vi "WPI_ADI_IMU_IMUAccumulation.vi"(1 "Input Data":T1) -> (0 "Output Data":T1)   [LabVIEW 2015, in "FRC ADI MXP IMU.lvlib"]
uses:
  FRC ADI MXP IMU.lvlib
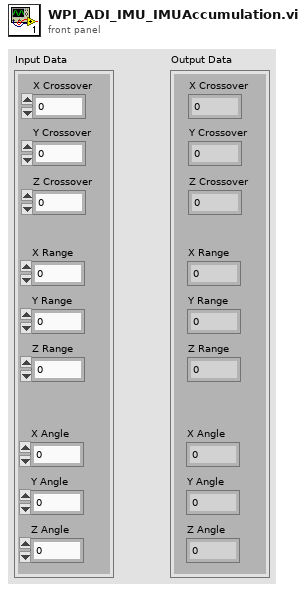
[diagram p1: front panel]
types:
  T1 = cluster{"X Crossover":dbl, "Y Crossover":dbl, "Z Crossover":dbl, "X Range":dbl, "Y Range":dbl, "Z Range":dbl, "X Angle":dbl, "Y Angle":dbl, "Z Angle":dbl}
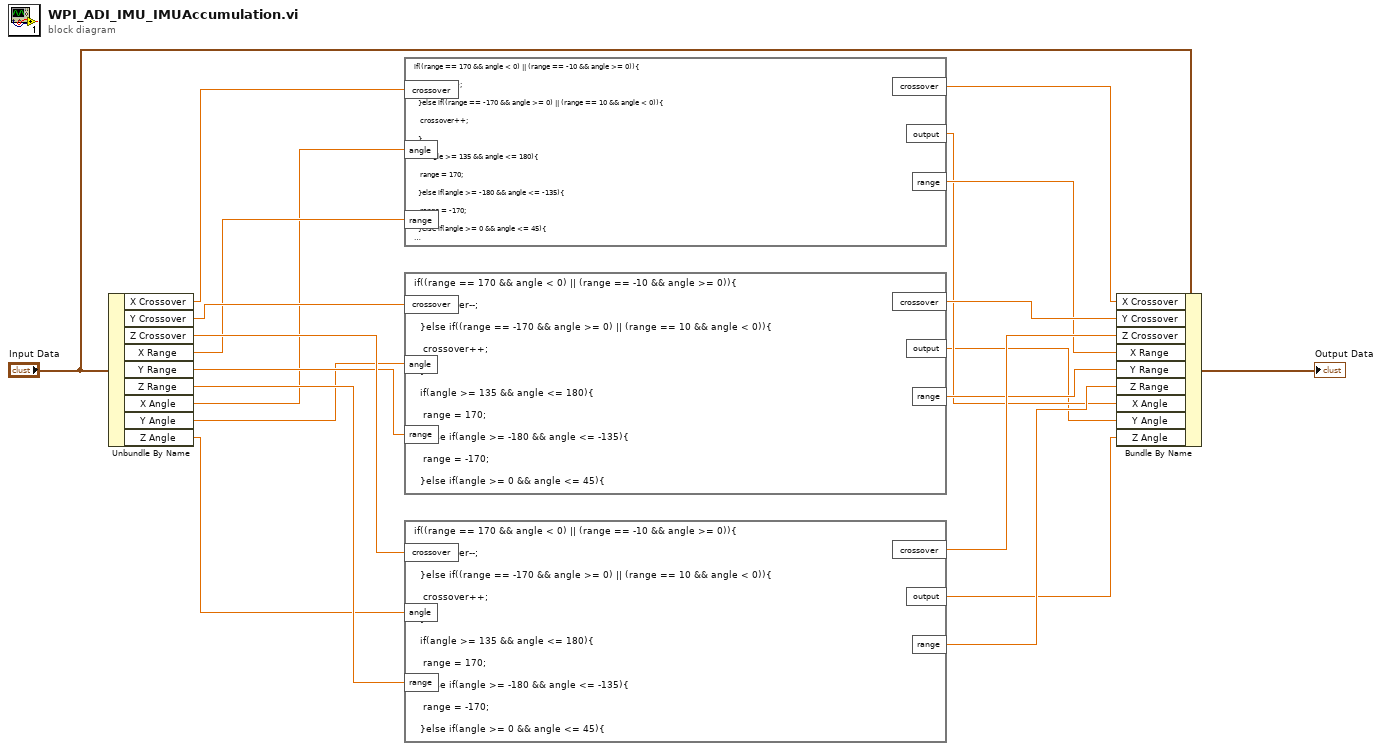
[diagram p0: block diagram]
diagram:
  n1 = Unbundle By Name("Input Data") -> ("X Crossover"=w20:dbl, "Y Crossover"=w19:dbl, "Z Crossover"=w18:dbl, "X Range"=w17:dbl, "Y Range"=w16:dbl, "Z Range"=w15:dbl, "X Angle"=w14:dbl, "Y Angle"=w13:dbl, "Z Angle"=w12:dbl)
  n2 = formula code="if((range == 170 && angle < 0) || (range == -10 && angle >= 0)){\n\t\t\n\t\t\tcrossover--;\n\t\t\t\n\t\t}else if((range == -170 && angle >= 0) || (range == 10 && angle < 0)){\n\t\t\n\t\t\tcrossover++;\n\t\t\t\n\t\t}\n\t\t\t\n\t\tif(angle >= 135 && angle <= 180){\n\t\t\n\t\t\trange = 170;\n\t\t\t\n\t\t}else if(angle >= -180 && angle <= -135){\n\t\t\n\t\t\trange = -170;\n\t\t\t\n\t\t}else if(angle >= 0 && angle <= 45){\n\t\t\n\t\t\trange = 10;\n\t\t\t\n\t\t}else if(angle >= -45 && angle <= 0){\n\t\t\n\t\t\trange = -10;\n\t\t\t\n\t\t}else{\n\t\t\n\t\t\trange = 0;\n\t\t\t\n\t\t}\n\t\t\n\t\tif(crossover != 0){\n\t\t\n\t\t\tif(angle < 0){\n\t\t\t\n\t\t\t\toutput = abs(180 + angle) + (-180 * crossover);\n\t\t\t\n\t\t\t}else{\n\t\t\n\t\t\t\toutput = abs(0 - angle) + (-180 * crossover);\n\t\t\n\t\t\t}\n\t\t\n\t\t}else{\n\t\t\n\t\t\toutput = angle;\n\t\t\n\t\t}"("crossover"=w20, "angle"=w14, "range"=w17) -> ("crossover"=w10:dbl, "output"=w4:dbl, "range"=w7:dbl)
  n3 = formula code="if((range == 170 && angle < 0) || (range == -10 && angle >= 0)){\n\t\t\n\t\t\tcrossover--;\n\t\t\t\n\t\t}else if((range == -170 && angle >= 0) || (range == 10 && angle < 0)){\n\t\t\n\t\t\tcrossover++;\n\t\t\t\n\t\t}\n\t\t\t\n\t\tif(angle >= 135 && angle <= 180){\n\t\t\n\t\t\trange = 170;\n\t\t\t\n\t\t}else if(angle >= -180 && angle <= -135){\n\t\t\n\t\t\trange = -170;\n\t\t\t\n\t\t}else if(angle >= 0 && angle <= 45){\n\t\t\n\t\t\trange = 10;\n\t\t\t\n\t\t}else if(angle >= -45 && angle <= 0){\n\t\t\n\t\t\trange = -10;\n\t\t\t\n\t\t}else{\n\t\t\n\t\t\trange = 0;\n\t\t\t\n\t\t}\n\t\t\n\t\tif(crossover != 0){\n\t\t\n\t\t\tif(angle < 0){\n\t\t\t\n\t\t\t\toutput = abs(180 + angle) + (-180 * crossover);\n\t\t\t\n\t\t\t}else{\n\t\t\n\t\t\t\toutput = abs(0 - angle) + (-180 * crossover);\n\t\t\n\t\t\t}\n\t\t\n\t\t}else{\n\t\t\n\t\t\toutput = angle;\n\t\t\n\t\t}"("crossover"=w19, "angle"=w13, "range"=w16) -> ("crossover"=w9:dbl, "output"=w2:dbl, "range"=w6:dbl)
  n4 = formula code="if((range == 170 && angle < 0) || (range == -10 && angle >= 0)){\n\t\t\n\t\t\tcrossover--;\n\t\t\t\n\t\t}else if((range == -170 && angle >= 0) || (range == 10 && angle < 0)){\n\t\t\n\t\t\tcrossover++;\n\t\t\t\n\t\t}\n\t\t\t\n\t\tif(angle >= 135 && angle <= 180){\n\t\t\n\t\t\trange = 170;\n\t\t\t\n\t\t}else if(angle >= -180 && angle <= -135){\n\t\t\n\t\t\trange = -170;\n\t\t\t\n\t\t}else if(angle >= 0 && angle <= 45){\n\t\t\n\t\t\trange = 10;\n\t\t\t\n\t\t}else if(angle >= -45 && angle <= 0){\n\t\t\n\t\t\trange = -10;\n\t\t\t\n\t\t}else{\n\t\t\n\t\t\trange = 0;\n\t\t\t\n\t\t}\n\t\t\n\t\tif(crossover != 0){\n\t\t\n\t\t\tif(angle < 0){\n\t\t\t\n\t\t\t\toutput = abs(180 + angle) + (-180 * crossover);\n\t\t\t\n\t\t\t}else{\n\t\t\n\t\t\t\toutput = abs(0 - angle) + (-180 * crossover);\n\t\t\n\t\t\t}\n\t\t\n\t\t}else{\n\t\t\n\t\t\toutput = angle;\n\t\t\n\t\t}"("crossover"=w18, "angle"=w12, "range"=w15) -> ("crossover"=w8:dbl, "output"=w3:dbl, "range"=w5:dbl)
  n5 = Bundle By Name(cluster="Input Data", "X Crossover"=w10, "Y Crossover"=w9, "Z Crossover"=w8, "X Range"=w7, "Y Range"=w6, "Z Range"=w5, "X Angle"=w4, "Y Angle"=w2, "Z Angle"=w3) -> (→"Output Data":T1)
